vi "Image Input.vi"() -> ()   [LabVIEW 2021]
panel:
  in  "Python version":string="3.9"
  in  "function name":string="predict_grade"
  in  "Python path":path=path "C:/Users/river/AppData/Local/Programs/Python/Python39/python.exe"
  out "OUTPUT GRADE":i32=1
  in  "module path":path=path "D:/9th/LabVIEW/testing/function.py"
  out "error out 3":errorcluster
  in  "stop":bool
  out "error out 2":errorcluster
  out "error out":errorcluster
  out "input":T1(plugin-control)
  in  "image Path":path=path "D:/9th/LabVIEW/testing/test_image2.jpeg"
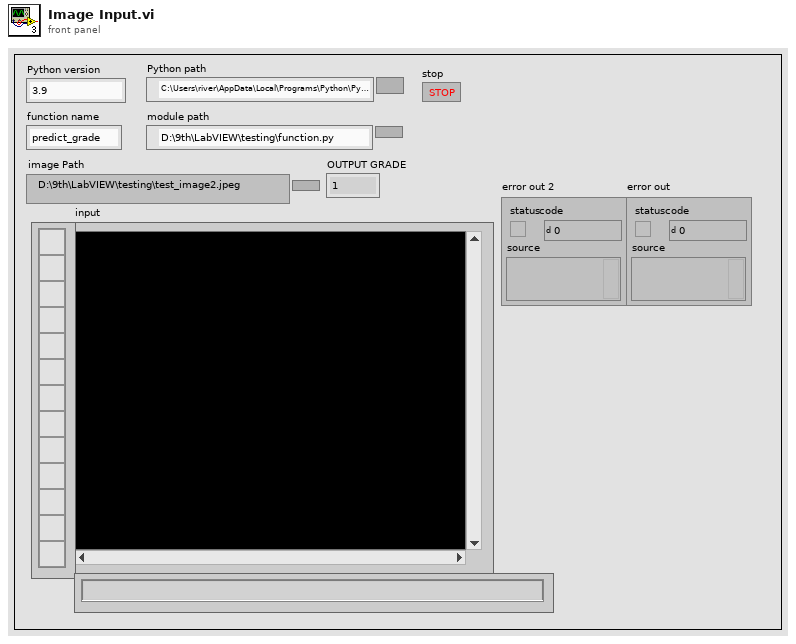
[diagram p1: front panel]
types:
  T1 = typedef "IMAQ Image.ctl" = refnum<image>
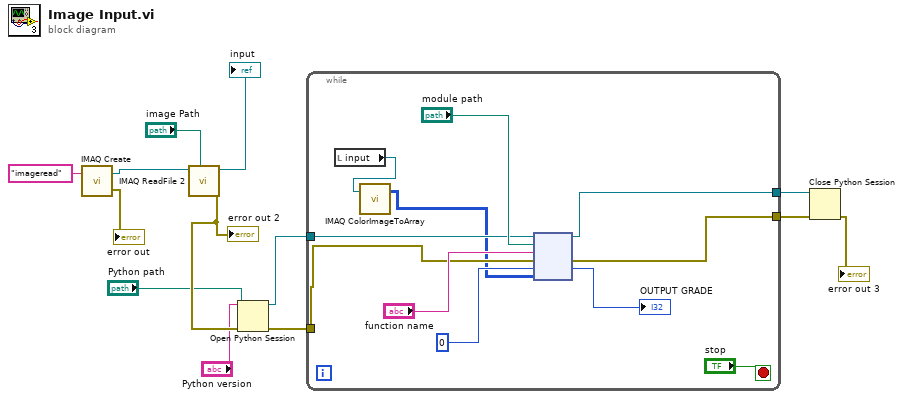
[diagram p0: block diagram]
diagram:
  n1 = call "IMAQ Create"("Image Name"="imageread") -> ("New Image"=w11:T1, "error out"=→"error out":errorcluster)  [unwired: 4 in]
  n2 = call "IMAQ ReadFile 2"("File Path"="image Path", "Image"=w11) -> ("error out"=w9:errorcluster, "Image Out"=→"input":T1)  [unwired: 5 in, 3 out]
  "error out 2" <- w9
  n3 = Open Python Session(python version="Python version", python path="Python path", 3:w9) -> (session out=w7:refnum<k35>, error out=w6:errorcluster)
  n4 = while {
    tunnel: w7 -> [w19]
    tunnel: w6 -> [w18]
    tunnel: [w17] -> w4
    tunnel: [w16] -> w3
    stop <- "stop" stop-if-true
    n5 = local read "input"() -> (w22:T1)
    n6 = call "IMAQ ColorImageToArray"("Image"=w22) -> ("Image Pixels (U32)"=w14:u32[][])  [unwired: 3 in, 2 out]
    n7 = node(w19, "module path", "function name", w18, 0 ("Numeric"), w14) -> (w17:refnum<k35>, w16:errorcluster, →"OUTPUT GRADE":i32)  [unwired: 1 in, 2 out]
  }
  n8 = Close Python Session(session in=w4, error in=w3) -> (11:→"error out 3":errorcluster)
